vi "Init Graph.vi"(4 "Z Scale.Marker Values[]":cluster{"Numeric":dbl, "Numeric":u32}[](array[cluster]), 6 "X-Graph Ref":refnum<vi>, 7 "Y-Graph Ref":refnum<vi>, 8 "error in (no error)":errorcluster, 9 "Images Size":cluster{"Height":u32, "Width":u32}, 10 "IntGraph Ref":refnum<vi>, 11 "Intensity Graph in":refnum<class "TG Graph.lvclass">) -> (0 "error out":errorcluster, 3 "Intensity Graph out":refnum<class "TG Graph.lvclass">)   [LabVIEW 2023, in "TG Graph.lvclass"]
uses:
  TG Graph.lvclass
  TG Graph.lvclass/TG Graph.ctl
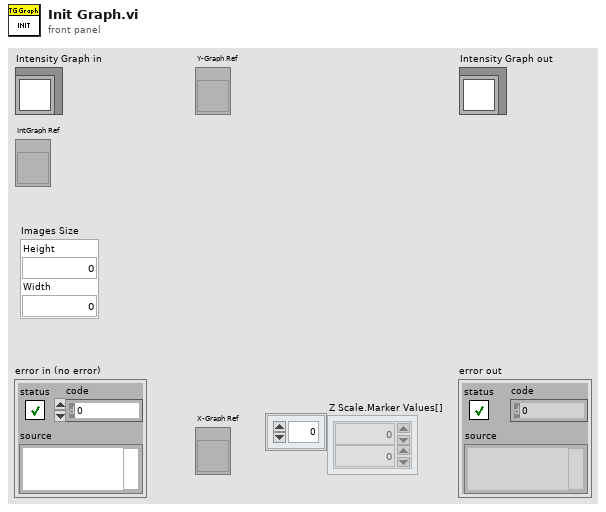
[diagram p1: front panel]
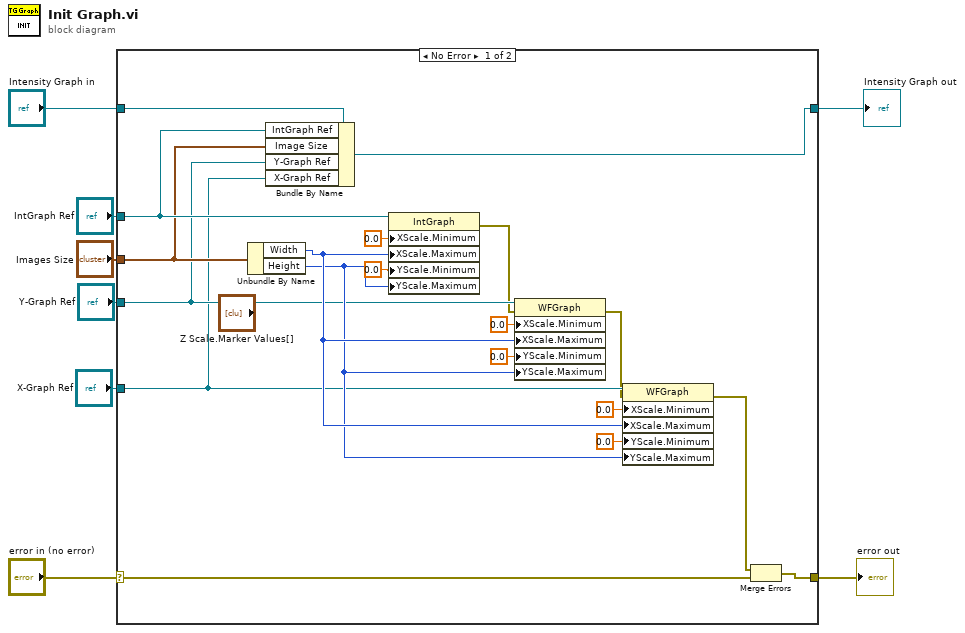
[diagram p0: block diagram]
diagram:
  n1 = case shown="No Error" "error in (no error)" {
    selector: "error in (no error)" -> [w27 w29]
    tunnel: [w13 w29] -> w7
    tunnel: [w12 w28] -> w5
    tunnel: "Intensity Graph in" -> [w18 w28]
    tunnel: "IntGraph Ref" -> [w17 _]
    tunnel: "Y-Graph Ref" -> [w15 _]
    tunnel: "X-Graph Ref" -> [w14 _]
    tunnel: "Images Size" -> [w16 _]
    frame No Error {
      n2 = Unbundle By Name(w16) -> ("Width"=w20:u32, "Height"=w19:u32)
      n3 = Bundle By Name(cluster=w18, "IntGraph Ref"=w17, "Image Size"=w16, "Y-Graph Ref"=w15, "X-Graph Ref"=w14) -> (w12:refnum<class "TG Graph.lvclass">)
      n4 = property class="IntGraph"(reference=w17, "XScale.Minimum"=0.0 ("X Scale.Range:Minimum"), "XScale.Maximum"=w20, "YScale.Minimum"=0.0 ("Y Scale.Range:Minimum"), "YScale.Maximum"=w19) -> (error out=w9:errorcluster)  [unwired: 1 in, 1 out]
      n5 = property class="WFGraph"(reference=w15, error in=w9, "XScale.Minimum"=0.0 ("X Scale.Range:Minimum"), "XScale.Maximum"=w20, "YScale.Minimum"=0.0 ("Y Scale.Range:Minimum"), "YScale.Maximum"=w19) -> (error out=w10:errorcluster)  [unwired: 1 out]
      n6 = property class="WFGraph"(reference=w14, error in=w10, "XScale.Minimum"=0.0 ("X Scale.Range:Minimum"), "XScale.Maximum"=w20, "YScale.Minimum"=0.0 ("Y Scale.Range:Minimum"), "YScale.Maximum"=w19) -> (error out=w11:errorcluster)  [unwired: 1 out]
      n7 = Merge Errors(w11, w27) -> (w13:errorcluster)
    }
    frame Error {
    }
  }
  "error out" <- w7
  "Intensity Graph out" <- w5
